vi "Write Num Nodes.vi"(8 "error in (no error)":errorcluster, 10 "Num Nodes":i32, 11 "abs_Composite in":refnum<class "bt_Composite.lvclass">) -> (0 "error out":errorcluster, 3 "abs_Composite out":refnum<class "bt_Composite.lvclass">)   [LabVIEW 2021, in "BT.lvlib" / "bt_Composite.lvclass"]
uses:
  bt_Composite.lvclass
  bt_Composite.lvclass/bt_Composite.ctl
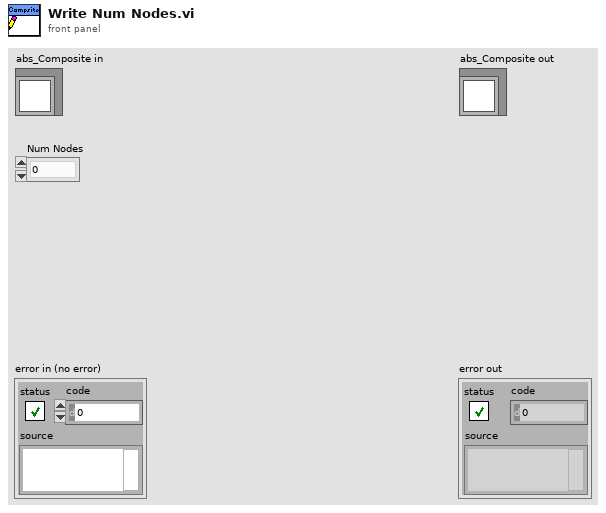
[diagram p1: front panel]
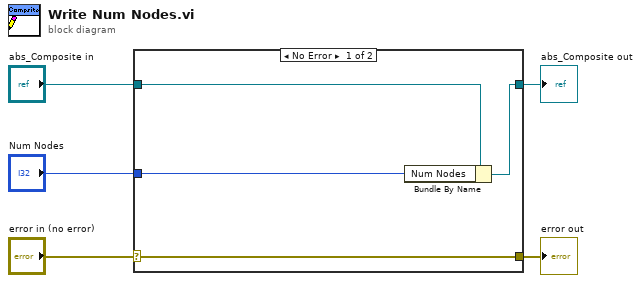
[diagram p0: block diagram]
diagram:
  n1 = case shown="No Error" "error in (no error)" {
    selector: "error in (no error)" -> [w9 w10]
    tunnel: [w9 w10] -> w4
    tunnel: [w7 w11] -> w2
    tunnel: "abs_Composite in" -> [w8 w11]
    tunnel: "Num Nodes" -> [w6 _]
    frame No Error {
      n2 = Bundle By Name(cluster=w8, "Num Nodes"=w6) -> (w7:refnum<class "bt_Composite.lvclass">)
    }
    frame Error {
    }
  }
  "error out" <- w4
  "abs_Composite out" <- w2
